vi "GetDC.vi"(8 "error in (no error)":errorcluster, 11 "hWnd":u32) -> (0 "error out":errorcluster, 3 "hdc":u32)   [LabVIEW 2019]
uses:
  user32.dll
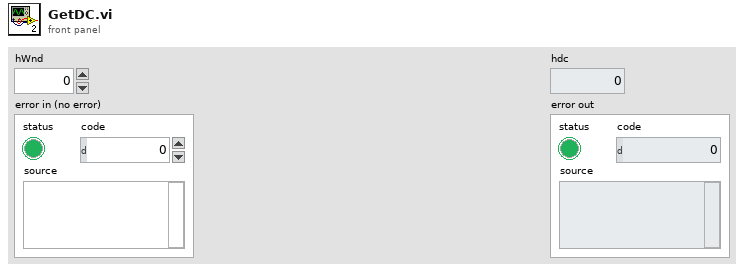
[diagram p1: front panel]
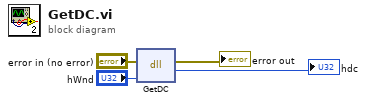
[diagram p0: block diagram]
diagram:
  n1 = dll-call lib="user32.dll" fn="GetDC"(error in="error in (no error)", "hWnd"="hWnd") -> (error out=→"error out":errorcluster, "hdc"=→"hdc":u32)  [unwired: 3 in, 1 out]
